vi "TDX Sim Data.vi"(10 "TDX in":sgl) -> (2 "TDX out":sgl)   [LabVIEW 2014, in "SimSyA.lvlib"]
uses:
  SimSyA.lvlib
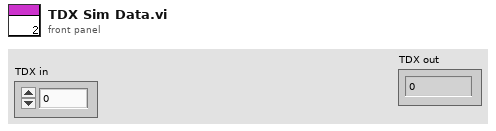
[diagram p1: front panel]
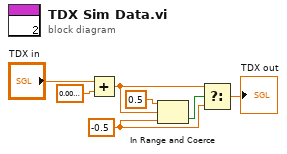
[diagram p0: block diagram]
diagram:
  w2 = sgl -0.5 ("lower limit")
  n1 = Add(x="TDX in", y=sgl 0.01) -> (x+y=w3:sgl)
  n2 = In Range and Coerce(upper limit=sgl 0.5, x=w3, lower limit=w2) -> (In Range?=w4:bool)  [unwired: 1 out]
  n3 = Select(t=w3, s=w4, f=w2) -> (s? t:f=→"TDX out":sgl)
